vi "Find DAQmx Digitizers.vi"(8 "Error In":errorcluster) -> (0 "Error Out":errorcluster, 2 "Device names":string[](array[string]), 3 "Digitizers out":refnum<class "Pulse Driver.lvclass">[](array[class]))   [LabVIEW 2019, in "DAQmx Synthesizer.lvclass"]
uses:
  DAQmx Synthesizer.lvclass
  Instruments/Pulse Driver/Pulse Driver.lvclass
  C:/github/NHMFL_Core/Libraries/Instruments/Pulse Driver/Pulse Driver.lvclass
  DAQmx Synthesizer.lvclass/DAQmx Synthesizer.ctl
  Write DAQmx Device Name.vi
  <resource>/objmgr/daqmx.rc
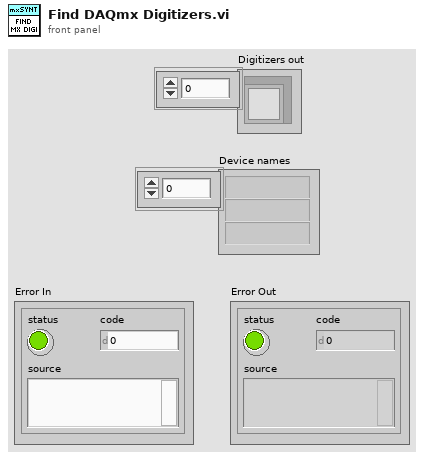
[diagram p1: front panel]
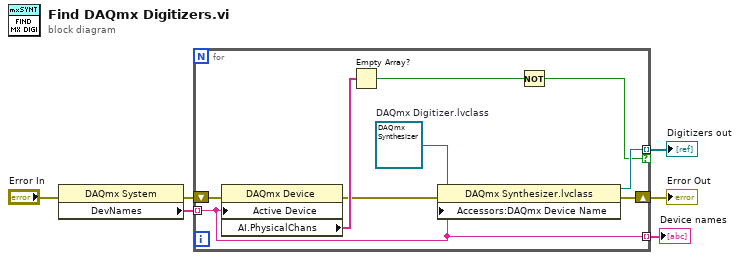
[diagram p0: block diagram]
diagram:
  n1 = property class="DAQmx System"(error in="Error In") -> (error out=w5:errorcluster, "DevNames"=w6:tag[])  [unwired: 1 in, 1 out]
  n2 = for {
    tunnel: w6 -> [w7] mode=indexing
    shift-right: [w11] -> w2
    shift-left: w5 -> [w15]
    tunnel: [w10] -> w3 mode=indexing if=w8
    tunnel: [w7] -> w1 mode=indexing
    w13 = refnum<class "DAQmx Synthesizer.lvclass"> refnum  # DAQmx Digitizer.lvclass
    n3 = property class="DAQmx Device"(error in=w15, "Active Device"=w7) -> (error out=w12:errorcluster, "AI.PhysicalChans"=w14:tag[])  [unwired: 1 in, 1 out]
    n4 = Empty Array?(array=w14) -> (empty?=w9:bool)
    n5 = property class="DAQmx Synthesizer.lvclass"(reference=w13, error in=w12, "Accessors:DAQmx Device Name"=w7) -> (reference out=w10:refnum<class "DAQmx Synthesizer.lvclass">, error out=w11:errorcluster)
    n6 = Not(x=w9) -> (.not. x?=w8:bool)
  }
  "Error Out" <- w2
  "Digitizers out" <- w3
  "Device names" <- w1
